vi "RT Main v0.82.vi"() -> ()   [LabVIEW 2017]
uses:
  Controls/Auto Delays.ctl
  support/Controls/All Inputs.ctl
  support/Controls/Index Details.ctl
  Global Variables/RT GV.vi
  support/Message Queue/Enqueue Message (Single).vi
  <vilib>/Utility/error.llb/Error Cluster From Error Code.vi
  <vilib>/rvi/errors/niLvFpgaAdjustHostInterfaceError.vi
  Global Variables/FPGA GV.vi
  Global Variables/Network Globals.vi
  <vilib>/FPGAPlugInAG/Dynamic/niLvFpga_Close_Dynamic.vi
  <vilib>/rvi/interface/nirviReadWriteControl/nirviReadWriteControl.xnode
  Controls/FPGA Ref.ctl
  <vilib>/rvi/interface/nirviCloseFPGA/nirviCloseFPGA.xnode
  support/Message Queue/Message Queue.lvlib
  NiFpgaLv.dll
  <vilib>/rvi/interface/Simulation/niFpgaSimulationCallBeginRW.vi
panel:
  in  "Auto Para":T1={"Agitator Delays"=[400, 250], "TF Delays"=[700, 800, 2], "Insertion Delays"=[100, 500], "Cutting Delays"=[300, 300, 100], "PF Delays"=[250, 30000], "Measur. Delays"=[500.0, 188.9, 1.0], "Reject Delays"=[500], "BF Delays"=[1000, 1000]}
  in  "Counts in":cluster{"OutputCount":u32, "RejectCount":u32}
  in  "Stop Button 4":bool
  in  "Stop Button 3":bool
  in  "Stop Button 2":bool
  out "error out":errorcluster
  out "Wrong Message":string
  in  "Stop Button":bool
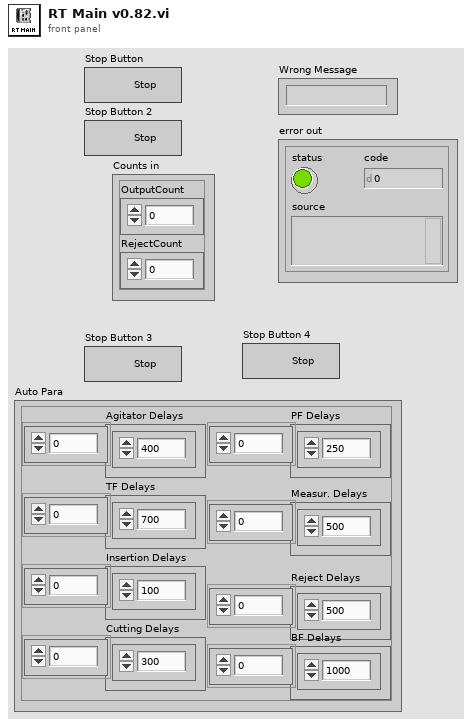
[diagram p1: front panel]
types:
  T1 = typedef "Auto Delays.ctl" = cluster{"Agitator Delays":u32[], "TF Delays":u32[], "Insertion Delays":u32[], "Cutting Delays":u32[], "PF Delays":u32[], "Measur. Delays":dbl[], "Reject Delays":u32[], "BF Delays":u32[]}
  T2 = typedef "FPGA Ref.ctl" = refnum<k20>
  T3 = cluster{"TL_Red":bool, "TL_Orange":bool, "TL_Green":bool, "TL_Buzzer":bool, "SOL_Index_Rotary_CW":bool, "SOL_Index_CNVR_Rotary_CCW":bool, "SOL_Index_CNVR_Stopper_Rear":bool, "SOL_Index_CNVR_Output _Separator _Rear":bool, "Bowl  Feeder_ ON":bool, "Pump_CNVR_Motor _ON":bool, "SOL_Gating_CYL_Rear":bool, "SOL_Tube_Feed_Agitatator":bool, "SOL_Tube_Feed_Gating_CYL":bool, "SOL_Insertion _CYL":bool, "SOL_Insertion_Clamp_CYL":bool, "SOL_Cutting_CYL":bool, "SOL_Cutting_Clamp_CYL":bool, "SOL_Insertion_Air_Nozzle":bool, "SOL_Measurement_CYL":bool, "SOL_Measure_Clamp_CYL":bool, "SOL_Rejection CYL_1":bool, "SOL_Rejection CYL_2":bool, "SOL_Rejection CYL_3":bool, "SOL_Rejection CYL_4":bool, "DO1.24":bool, "DO1.25":bool, "DO1.26":bool, "DO1.27":bool, "DO1.28":bool, "DO1.29":bool, "DO1.30":bool, "DO1.31":bool}
  T4 = typedef "All Inputs.ctl" = cluster{"DI 1":cluster{"Machine_ON":bool, "E_stop ":bool, "SW_Pressure":bool, "SW_Start ":bool, "SW_Reset":bool, "SW_Stop":bool, "SW_Door":bool, "RS_Index_Rotary_CW":bool, "RS_Index_Rotary_CCW":bool, "RS_Index_Stopper _Rear":bool, "RS_Index_Output_Separator_Rear":bool, "PES_Index_Pallet_Sensor":bool, "PES_Index_Output_Part Sensor":bool, "ICS_BF_Low_Level_1":bool, "ICS_BF_Low_Level_2":bool, "ICS_BF_Pump_CNVR_Full_1":bool, "ICS_BF_Pump_CNVR_Full_2":bool, "ICS_BF_Pump_CNVR_Full_3":bool, "ICS_BF_Pump_CNVR_Full_4":bool, "PES_PC_Pump Presence_1":bool, "PES_PC_Pump Presence_2":bool, "PES_PC_Pump Presence_3":bool, "PES_PC_Pump Presence_4":bool, "RS_PC_Gating_Front":bool, "PES_Pump_Interference":bool, "PES_TF_Low_Level":bool, "PES_Tube Presence_1":bool, "PES_Tube Presence_2":bool, "PES_Tube Presence_3":bool, "PES_Tube Presence_4":bool, "DI1.30":bool, "DI1.31":bool}, "DI 2":cluster{"RS_Agitatator_1_Rear ":bool, "RS_Agitatator_2_Rear ":bool, "RS_TF_Gating CYL_Rear":bool, "RS_Insertion_1_Rear":bool, "RS_Insertion_1_Front":bool, "RS_Insertion _2_Rear":bool, "RS_Insertion _2_Front":bool, "RS_Insertion _3_Rear":bool, "RS_Insertion _3_Front":bool, "RS_Insertion _4_Rear":bool, "RS_Insertion _4_Front":bool, "RS_Insertion_Clamp_Rear":bool, "RS_Cutting_Rear":bool, "RS_Cutting_Clamp _Rear":bool, "RS_Measurement_1_Rear":bool, "RS_Measurement_2_Rear":bool, "RS_Measurement_3_Rear":bool, "RS_Measurement_4_Rear":bool, "RS_Measure_Clamp_Rear":bool, "RS_Rejection_1_Rear":bool, "RS_Rejection_2_Rear":bool, "RS_Rejection_3_Rear":bool, "RS_Rejection_4_Rear":bool, "DI2.23":bool, "DI2.24":bool, "DI2.25":bool, "DI2.26":bool, "DI2.27":bool, "DI2.28":bool, "DI2.29":bool, "DI2.30":bool, "DI2.31":bool}, "IAS 1":dbl, "IAS 2":dbl, "IAS 3":dbl, "IAS 4":dbl, "DO 1":cluster{"TL_Red":bool, "TL_Orange":bool, "TL_Green":bool, "TL_Buzzer":bool, "SOL_Index_Rotary_CW":bool, "SOL_Index_CNVR_Rotary_CCW":bool, "SOL_Index_CNVR_Stopper_Rear":bool, "SOL_Index_CNVR_Output _Separator _Rear":bool, "Bowl  Feeder_ ON 1":bool, "Pump_CNVR_Motor _ON":bool, "SOL_PC_Gating_CYL_Rear":bool, "SOL_Tube_Feed_Agitatator":bool, "SOL_Tube_Feed_Gating_CYL":bool, "SOL_Insertion _CYL":bool, "SOL_Insertion_Clamp_CYL":bool, "SOL_Cutting_CYL":bool, "SOL_Cutting_Clamp_CYL":bool, "SOL_Insertion_Air_Nozzle":bool, "SOL_Measurement_CYL":bool, "DO1.19":bool, "SOL_Rejection CYL_1":bool, "SOL_Rejection CYL_2":bool, "SOL_Rejection CYL_3":bool, "SOL_Rejection CYL_4":bool, "Bowl  Feeder_ ON 2":bool, "SOL_BF_BlowerON":bool, "SOL_BF1_Track1":bool, "SOL_BF1_Track2":bool, "SOL_BF2_Track1":bool, "SOL_BF2_Track2":bool, "DO1.30":bool, "DO1.31":bool}}
  T5 = typedef "Index Details.ctl" = cluster{"Time (ms)":u32, "Waveform Graph":i16[]}
  T6 = cluster{T1, "Reject Pallets":cluster{"Reject 1":bool, "Reject 2":bool, "Reject 3":bool, "Reject 4":bool}}
  T7 = cluster{string, dbl, "Counts in":cluster{"OutputCount":u32, "RejectCount":u32}, "Auto Para":T1}
  T8 = cluster{"TL_Red":bool, "TL_Orange":bool, "TL_Green":bool, "TL_Buzzer":bool, "SOL_Index_Rotary_CW":bool, "SOL_Index_CNVR_Rotary_CCW":bool, "SOL_Index_CNVR_Stopper_Rear":bool, "SOL_Index_CNVR_Output _Separator _Rear":bool, "Bowl Feeder_ ON1":bool, "Pump_CNVR_Motor _ON":bool, "SOL_PC_Gating_CYL_Rear":bool, "SOL_Tube_Feed_Agitatator":bool, "SOL_Tube_Feed_Gating_CYL":bool, "SOL_Insertion _CYL":bool, "SOL_Insertion_Clamp_CYL":bool, "SOL_Cutting_CYL":bool, "SOL_Cutting_Clamp_CYL":bool, "SOL_Insertion_Air_Nozzle":bool, "SOL_Measurement_CYL":bool, "DO1.19":bool, "SOL_Rejection CYL_1":bool, "SOL_Rejection CYL_2":bool, "SOL_Rejection CYL_3":bool, "SOL_Rejection CYL_4":bool, "Bowl Feeder_ON2":bool, "SOL_BF_BlowerON":bool, "SOL_BF1_Track1":bool, "SOL_BF1_Track2":bool, "SOL_BF2_Track1":bool, "SOL_BF2_Track2":bool, "DO1.30":bool, "DO1.31":bool}
  T9 = cluster{"Machine_ON":bool, "E_stop ":bool, "SW_Pressure":bool, "SW_Start ":bool, "SW_Reset":bool, "SW_Stop":bool, "SW_Door":bool, "RS_Index_Rotary_CW":bool, "RS_Index_Rotary_CCW":bool, "RS_Index_Stopper _Rear":bool, "RS_Index_Output_Separator_Rear":bool, "PES_Index_Pallet_Sensor":bool, "PES_Index_Output_Part Sensor":bool, "ICS_BF_Low_Level_1":bool, "ICS_BF_Low_Level_2":bool, "ICS_BF_Pump_CNVR_Full_1":bool, "ICS_BF_Pump_CNVR_Full_2":bool, "ICS_BF_Pump_CNVR_Full_3":bool, "ICS_BF_Pump_CNVR_Full_4":bool, "PES_PC_Pump Presence_1":bool, "PES_PC_Pump Presence_2":bool, "PES_PC_Pump Presence_3":bool, "PES_PC_Pump Presence_4":bool, "RS_PC_Gating_Front":bool, "PES_Pump_Interference":bool, "PES_TF_Low_Level":bool, "PES_Tube Presence_1":bool, "PES_Tube Presence_2":bool, "PES_Tube Presence_3":bool, "PES_Tube Presence_4":bool, "DI1.30":bool, "DI1.31":bool}
  T10 = cluster{"RS_Agitatator_1_Rear ":bool, "RS_Agitatator_2_Rear ":bool, "RS_TF_Gating CYL_Rear":bool, "RS_Insertion_1_Rear":bool, "RS_Insertion_1_Front":bool, "RS_Insertion _2_Rear":bool, "RS_Insertion _2_Front":bool, "RS_Insertion _3_Rear":bool, "RS_Insertion _3_Front":bool, "RS_Insertion _4_Rear":bool, "RS_Insertion _4_Front":bool, "RS_Insertion_Clamp_Rear":bool, "RS_Cutting_Rear":bool, "RS_Cutting_Clamp _Rear":bool, "RS_Measurement_1_Rear":bool, "RS_Measurement_2_Rear":bool, "RS_Measurement_3_Rear":bool, "RS_Measurement_4_Rear":bool, "DI2.18":bool, "RS_Rejection_1_Rear":bool, "RS_Rejection_2_Rear":bool, "RS_Rejection_3_Rear":bool, "RS_Rejection_4_Rear":bool, "DI2.23":bool, "DI2.24":bool, "DI2.25":bool, "DI2.26":bool, "DI2.27":bool, "DI2.28":bool, "DI2.29":bool, "DI2.30":bool, "DI2.31":bool}
  T11 = cluster{"Measurements":cluster{"1":dbl, "2":dbl, "3":dbl, "4":dbl}, "Reject Pallets":cluster{"Reject 1":bool, "Reject 2":bool, "Reject 3":bool, "Reject 4":bool}}
  T12 = typedef "Auto Times.ctl" = cluster{"Index Time":u32, "TF Time":u32, "Insertion Time":u32, "Cutting Time":u32, "PF Time":u32, "Meas. Time":u32, "Reject Time":u32}
  T13 = cluster{"Auto Times":T12, "Results":cluster{"Measurements":cluster{"1":dbl, "2":dbl, "3":dbl, "4":dbl}, "Reject Pallets":cluster{"Reject 1":bool, "Reject 2":bool, "Reject 3":bool, "Reject 4":bool}}, "OutputCount":u32, "error out":errorcluster}
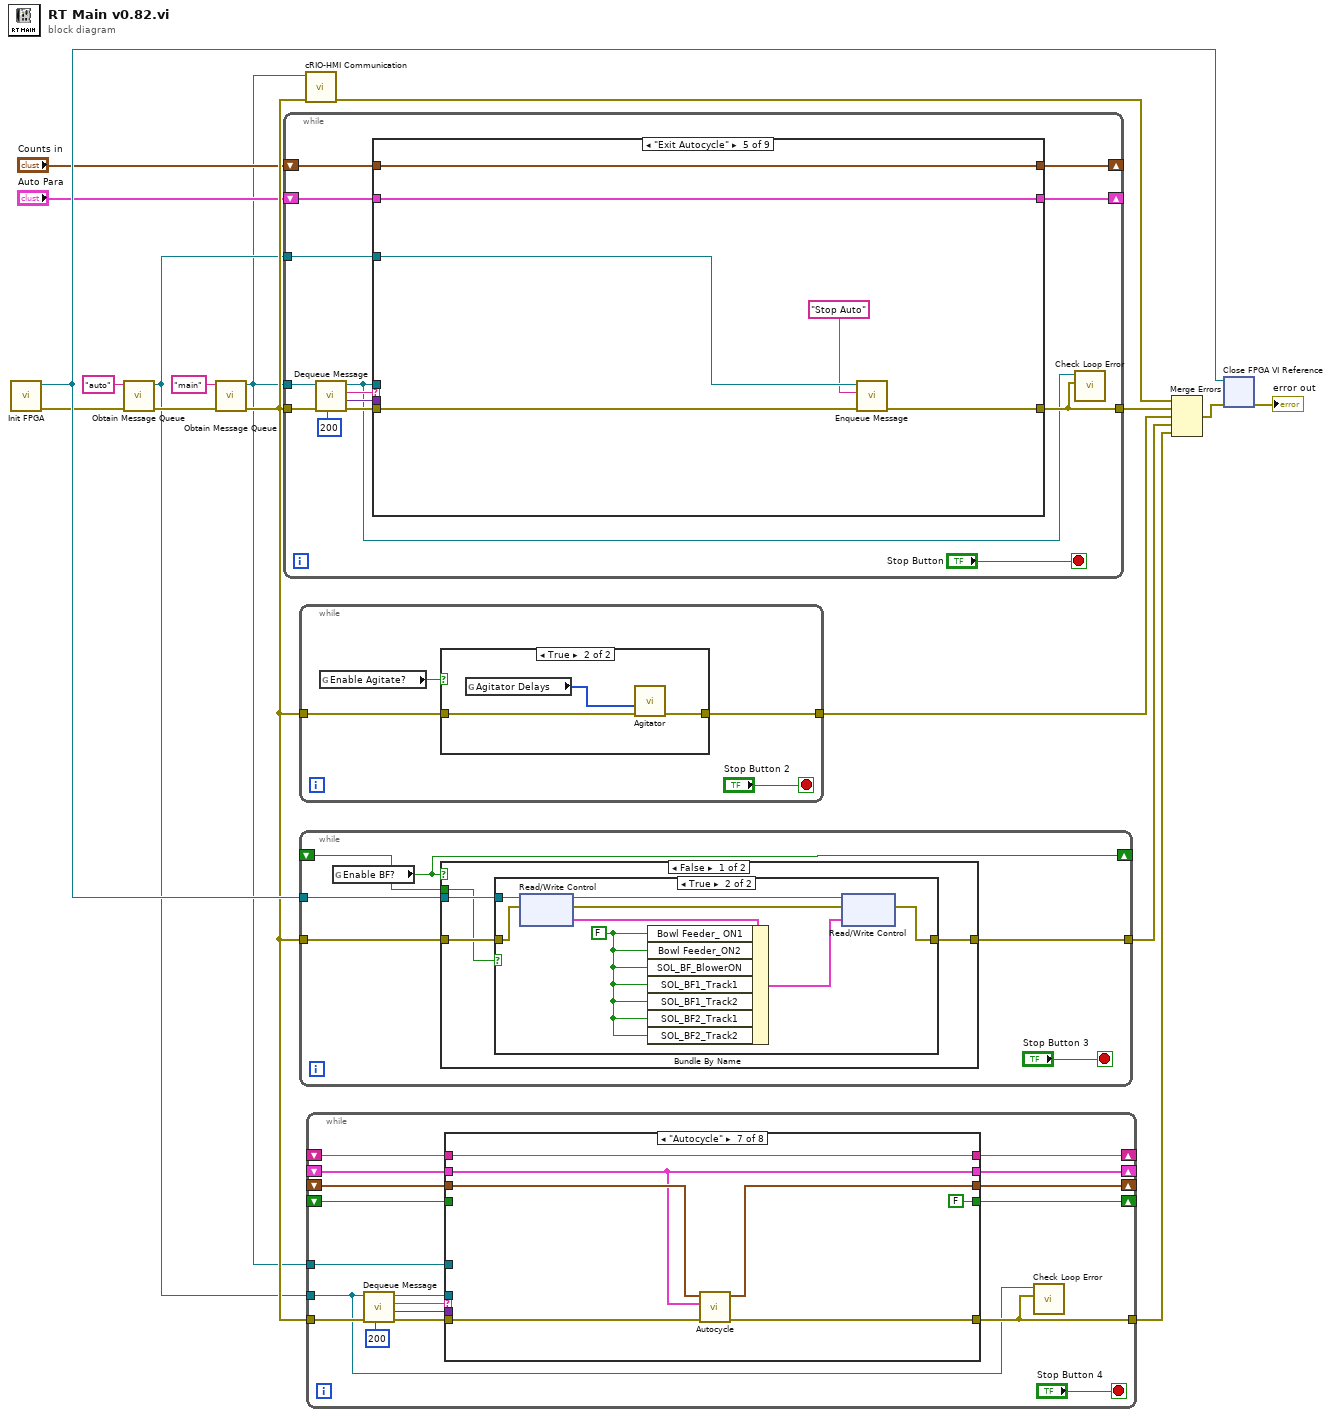
[diagram p0: block diagram]
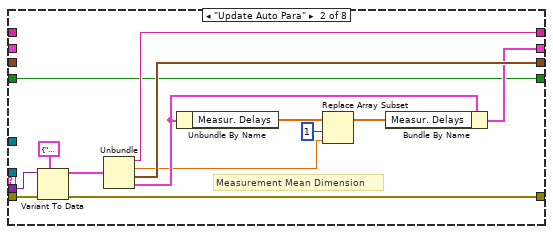
[diagram p3: hidden frame]
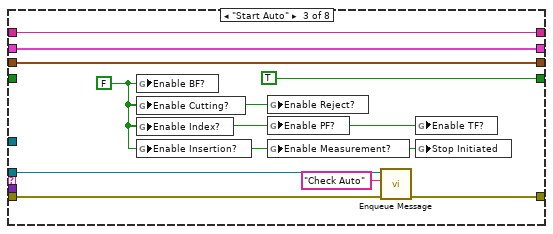
[diagram p4: hidden frame]
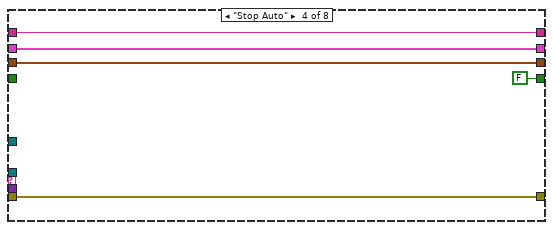
[diagram p5: hidden frame]
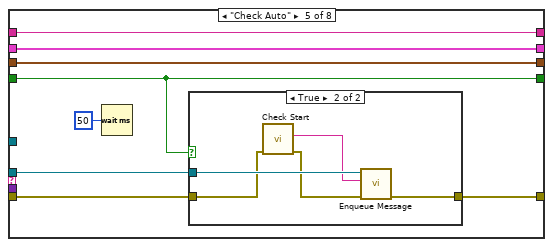
[diagram p6: hidden frame]
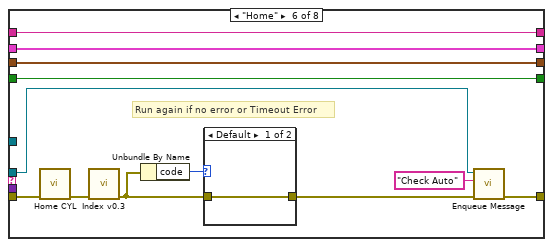
[diagram p8: hidden frame]
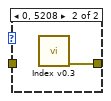
[diagram p9: hidden frame]
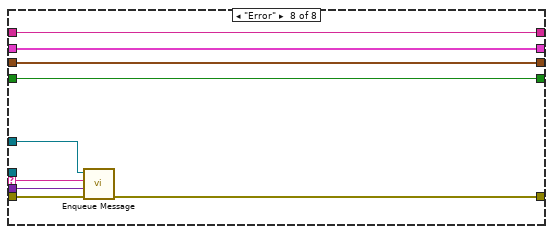
[diagram p10: hidden frame]
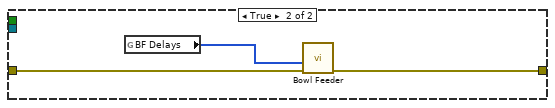
[diagram p12: hidden frame]
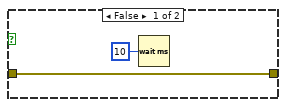
[diagram p13: hidden frame]
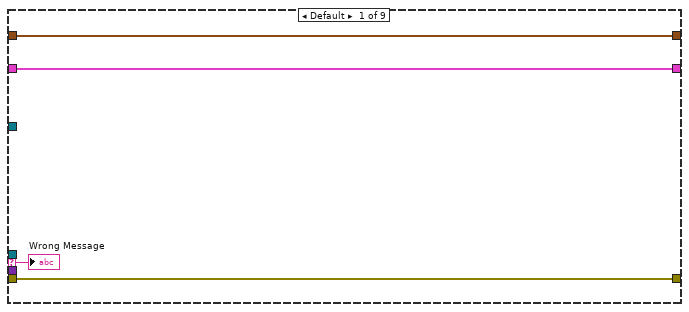
[diagram p14: hidden frame]
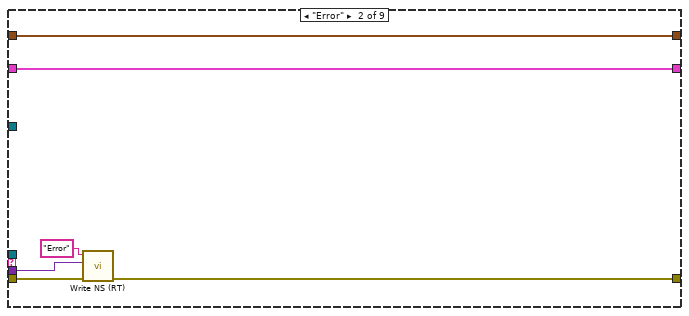
[diagram p15: hidden frame]
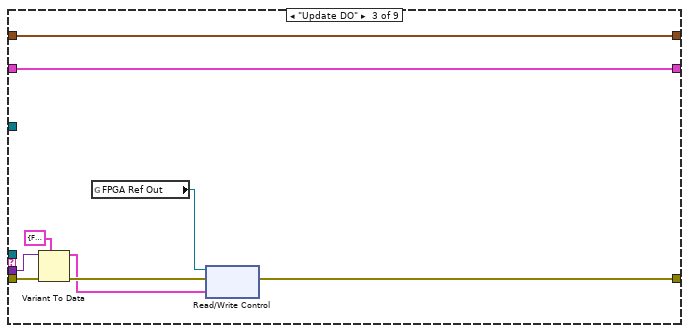
[diagram p16: hidden frame]
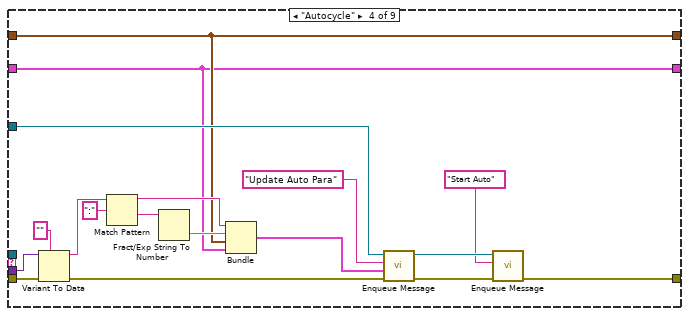
[diagram p17: hidden frame]
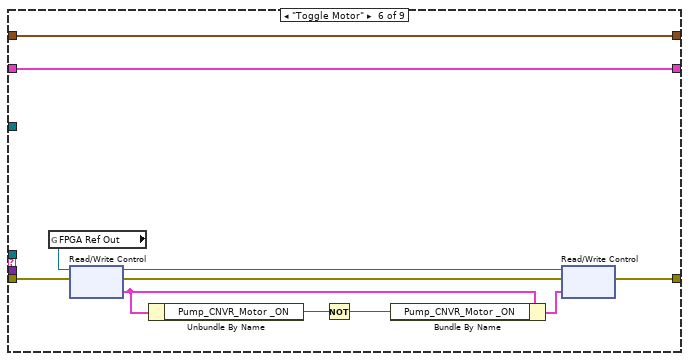
[diagram p18: hidden frame]
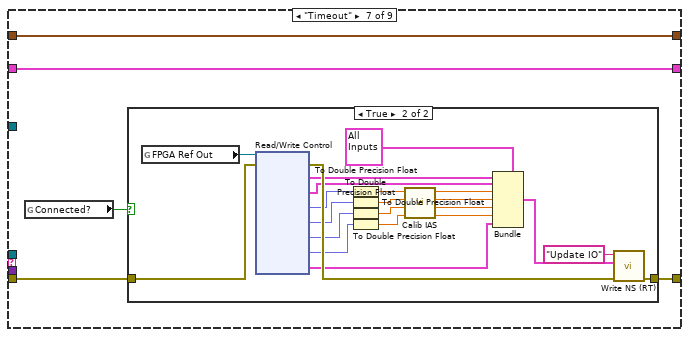
[diagram p19: hidden frame]
diagram:
  n1 = call "Init FPGA.vi"() -> ("error out"=w6:errorcluster, "FPGA Ref Out"=w11:T2)  [unwired: 10 in]
  n2 = call "Obtain Message Queue.vi"("error in (no error)"=w6, "name"="auto") -> ("error out"=w5:errorcluster, "Message Queue"=w2:refnum<queue>)  [unwired: 8 in]
  n3 = call "Obtain Message Queue.vi"("error in (no error)"=w5, "name"="main") -> ("error out"=w10:errorcluster, "Message Queue"=w1:refnum<queue>)  [unwired: 8 in]
  n4 = while {
    tunnel: w10 -> [w30]
    tunnel: w1 -> [w29]
    tunnel: [w25] -> w17
    tunnel: w2 -> [w22]
    shift-right: [w19] -> _
    shift-left: "Auto Para" -> [w20]
    shift-right: [w18] -> _
    shift-left: "Counts in" -> [w21]
    stop <- "Stop Button" stop-if-true
    n5 = call "Dequeue Message.vi"("timeout"=200, "error in (no error)"=w30, "Message Queue"=w29) -> ("error out"=w28:errorcluster, "Message Data"=w26:variant, "Message"=w27:string, "dup Message Queue"=w24:refnum<queue>)  [unwired: 5 in]
    n6 = case shown="\"Exit Autocycle\"" w27 {
      selector: w27 -> [w35 _ _ _ _ _ _ _ _]
      tunnel: w28 -> [w34 w39 w50 w68 w74 w84 w89 w125 w152]
      tunnel: w24 -> [_ _ _ _ _ _ _ w117 _]
      tunnel: w26 -> [_ w37 w49 w67 _ _ _ _ w151]
      tunnel: [w34 w38 w45 w53 w70 w82 w90 w118 w147] -> w25
      tunnel: w22 -> [_ _ _ w60 w73 _ _ _ _]
      tunnel: w21 -> [w33 w41 w43 w57 w72 w76 w87 w114 w138]
      tunnel: w20 -> [w32 w40 w42 w56 w71 w75 w86 w115 w137]
      tunnel: [w32 w40 w42 w56 w71 w75 w86 w115 w137] -> w19
      tunnel: [w33 w41 w43 w57 w72 w76 w87 w114 w138] -> w18
      frame Default {
        "Wrong Message" <- w35
      }
      frame "Error" {
        n7 = call "Write NS (RT).vi"("error in (no error)"=w39, "Message Data"=w37, "Message"="Error") -> ("error out"=w38:errorcluster)  [unwired: 8 in]
      }
      frame "Update DO" {
        n8 = Variant To Data(error in=w50, type=T3 {"TL_Red"=FALSE, "TL_Orange"=FALSE, "TL_Green"=FALSE, "TL_Buzzer"=FALSE, "SOL_Index_Rotary_CW"=FALSE, "SOL_Index_CNVR_Rotary_CCW"=FALSE, "SOL_Index_CNVR_Stopper_Rear"=FALSE, "SOL_Index_CNVR_Output _Separator _Rear"=FALSE, "Bowl  Feeder_ ON"=FALSE, "Pump_CNVR_Motor _ON"=FALSE, "SOL_Gating_CYL_Rear"=FALSE, "SOL_Tube_Feed_Agitatator"=FALSE, "SOL_Tube_Feed_Gating_CYL"=FALSE, "SOL_Insertion _CYL"=FALSE, "SOL_Insertion_Clamp_CYL"=FALSE, "SOL_Cutting_CYL"=FALSE, "SOL_Cutting_Clamp_CYL"=FALSE, "SOL_Insertion_Air_Nozzle"=FALSE, "SOL_Measurement_CYL"=FALSE, "SOL_Measure_Clamp_CYL"=FALSE, "SOL_Rejection CYL_1"=FALSE, "SOL_Rejection CYL_2"=FALSE, "SOL_Rejection CYL_3"=FALSE, "SOL_Rejection CYL_4"=FALSE, "DO1.24"=FALSE, "DO1.25"=FALSE, "DO1.26"=FALSE, "DO1.27"=FALSE, "DO1.28"=FALSE, "DO1.29"=FALSE, "DO1.30"=FALSE, "DO1.31"=FALSE} ("DO 1"), Variant=w49) -> (data=w44:T3, error out=w46:errorcluster)
        n9 = global read "FPGA GV.vi" "FPGA Ref Out"() -> (w47:T2)
        n10 = xnode "Read/Write Control"("FPGA VI Reference In"=w47, "error in"=w46, "DO 1"=w44) -> ("error out"=w45:errorcluster)  [unwired: 1 out]
      }
      frame "Autocycle" {
        n11 = Variant To Data(error in=w68, type="", Variant=w67) -> (data=w63:string, error out=w61:errorcluster)
        n12 = Match Pattern(string=w63, regular expression=":") -> (before substring=w59:string, after substring=w64:string)  [unwired: 1 in, 2 out]
        n13 = Fract/Exp String To Number(string=w64) -> (number=w58:dbl)  [unwired: 3 in, 1 out]
        n14 = Bundle(w59, w58, "Counts in"=w57, "Auto Para"=w56) -> (w55:T7)  [unwired: 1 in]
        n15 = call-poly "Enqueue Message.vi"("error in (no error)"=w61, "Message Data"=w55, "Message"="Update Auto Para", "Message Queue"=w60) -> ("error out"=w54:errorcluster, "dup Message Queue"=w52:refnum<queue>)  [unwired: 6 in]
        n16 = call-poly "Enqueue Message.vi"("error in (no error)"=w54, "Message"="Start Auto", "Message Queue"=w52) -> ("error out"=w53:errorcluster)  [unwired: 7 in, 1 out]
      }
      frame "Exit Autocycle" {
        n17 = call-poly "Enqueue Message.vi"("error in (no error)"=w74, "Message"="Stop Auto", "Message Queue"=w73) -> ("error out"=w70:errorcluster)  [unwired: 7 in, 1 out]
      }
      frame "Toggle Motor" {
        n18 = global read "FPGA GV.vi" "FPGA Ref Out"() -> (w85:T2)
        n19 = xnode "Read/Write Control"("FPGA VI Reference In"=w85, "error in"=w84) -> ("FPGA VI Reference Out"=w81:T2, "error out"=w83:errorcluster, "DO 1"=w79:T8)
        n20 = Unbundle By Name(w79) -> ("Pump_CNVR_Motor _ON"=w80:bool)
        n21 = Not(x=w80) -> (.not. x?=w77:bool)
        n22 = Bundle By Name(cluster=w79, "Pump_CNVR_Motor _ON"=w77) -> (w78:T8)
        n23 = xnode "Read/Write Control"("FPGA VI Reference In"=w81, "error in"=w83, "DO 1"=w78) -> ("error out"=w82:errorcluster)  [unwired: 1 out]
      }
      frame "Timeout" {
        n24 = global read "Network Globals.vi" "Connected?"() -> (w88:bool)
        n25 = case shown="True" w88 {
          tunnel: [w91 w112] -> w90
          tunnel: w89 -> [w91 w110]
          frame False {
          }
          frame True {
            n26 = global read "FPGA GV.vi" "FPGA Ref Out"() -> (w111:T2)
            n27 = xnode "Read/Write Control"("FPGA VI Reference In"=w111, "error in"=w110) -> ("error out"=w109:errorcluster, "DI 1"=w108:T9, "DI 2"=w107:T10, "AI0"=w106:fxp<+/-,27,6>, "AI1"=w105:fxp<+/-,27,6>, "AI2"=w104:fxp<+/-,27,6>, "AI3"=w103:fxp<+/-,27,6>, "DO 1"=w100:T8)  [unwired: 1 out]
            n28 = To Double Precision Float(number=w106) -> (double precision float=w93:dbl)
            n29 = To Double Precision Float(number=w105) -> (double precision float=w95:dbl)
            n30 = To Double Precision Float(number=w104) -> (double precision float=w97:dbl)
            n31 = To Double Precision Float(number=w103) -> (double precision float=w99:dbl)
            n32 = call "Calib IAS.vi"("x 4"=w99, "x 3"=w97, "x 2"=w95, "x"=w93) -> ("y 4"=w98:dbl, "y 3"=w96:dbl, "y 2"=w94:dbl, "y 1"=w92:dbl)  [unwired: 4 in]
            n33 = Bundle(cluster=T4 {"DI 1"={"Machine_ON"=FALSE, "E_stop "=FALSE, "SW_Pressure"=FALSE, "SW_Start "=FALSE, "SW_Reset"=FALSE, "SW_Stop"=FALSE, "SW_Door"=FALSE, "RS_Index_Rotary_CW"=FALSE, "RS_Index_Rotary_CCW"=FALSE, "RS_Index_Stopper _Rear"=FALSE, "RS_Index_Output_Separator_Rear"=FALSE, "PES_Index_Pallet_Sensor"=FALSE, "PES_Index_Output_Part Sensor"=FALSE, "ICS_BF_Low_Level_1"=FALSE, "ICS_BF_Low_Level_2"=FALSE, "ICS_BF_Pump_CNVR_Full_1"=FALSE, "ICS_BF_Pump_CNVR_Full_2"=FALSE, "ICS_BF_Pump_CNVR_Full_3"=FALSE, "ICS_BF_Pump_CNVR_Full_4"=FALSE, "PES_PC_Pump Presence_1"=FALSE, "PES_PC_Pump Presence_2"=FALSE, "PES_PC_Pump Presence_3"=FALSE, "PES_PC_Pump Presence_4"=FALSE, "RS_PC_Gating_Front"=FALSE, "PES_Pump_Interference"=FALSE, "PES_TF_Low_Level"=FALSE, "PES_Tube Presence_1"=FALSE, "PES_Tube Presence_2"=FALSE, "PES_Tube Presence_3"=FALSE, "PES_Tube Presence_4"=FALSE, "DI1.30"=FALSE, "DI1.31"=FALSE}, "DI 2"={"RS_Agitatator_1_Rear "=FALSE, "RS_Agitatator_2_Rear "=FALSE, "RS_TF_Gating CYL_Rear"=FALSE, "RS_Insertion_1_Rear"=FALSE, "RS_Insertion_1_Front"=FALSE, "RS_Insertion _2_Rear"=FALSE, "RS_Insertion _2_Front"=FALSE, "RS_Insertion _3_Rear"=FALSE, "RS_Insertion _3_Front"=FALSE, "RS_Insertion _4_Rear"=FALSE, "RS_Insertion _4_Front"=FALSE, "RS_Insertion_Clamp_Rear"=FALSE, "RS_Cutting_Rear"=FALSE, "RS_Cutting_Clamp _Rear"=FALSE, "RS_Measurement_1_Rear"=FALSE, "RS_Measurement_2_Rear"=FALSE, "RS_Measurement_3_Rear"=FALSE, "RS_Measurement_4_Rear"=FALSE, "RS_Measure_Clamp_Rear"=FALSE, "RS_Rejection_1_Rear"=FALSE, "RS_Rejection_2_Rear"=FALSE, "RS_Rejection_3_Rear"=FALSE, "RS_Rejection_4_Rear"=FALSE, "DI2.23"=FALSE, "DI2.24"=FALSE, "DI2.25"=FALSE, "DI2.26"=FALSE, "DI2.27"=FALSE, "DI2.28"=FALSE, "DI2.29"=FALSE, "DI2.30"=FALSE, "DI2.31"=FALSE}, "IAS 1"=0.0, "IAS 2"=0.0, "IAS 3"=0.0, "IAS 4"=0.0, "DO 1"={"TL_Red"=FALSE, "TL_Orange"=FALSE, "TL_Green"=FALSE, "TL_Buzzer"=FALSE, "SOL_Index_Rotary_CW"=FALSE, "SOL_Index_CNVR_Rotary_CCW"=FALSE, "SOL_Index_CNVR_Stopper_Rear"=FALSE, "SOL_Index_CNVR_Output _Separator _Rear"=FALSE, "Bowl  Feeder_ ON 1"=FALSE, "Pump_CNVR_Motor _ON"=FALSE, "SOL_PC_Gating_CYL_Rear"=FALSE, "SOL_Tube_Feed_Agitatator"=FALSE, "SOL_Tube_Feed_Gating_CYL"=FALSE, "SOL_Insertion _CYL"=FALSE, "SOL_Insertion_Clamp_CYL"=FALSE, "SOL_Cutting_CYL"=FALSE, "SOL_Cutting_Clamp_CYL"=FALSE, "SOL_Insertion_Air_Nozzle"=FALSE, "SOL_Measurement_CYL"=FALSE, "DO1.19"=FALSE, "SOL_Rejection CYL_1"=FALSE, "SOL_Rejection CYL_2"=FALSE, "SOL_Rejection CYL_3"=FALSE, "SOL_Rejection CYL_4"=FALSE, "Bowl  Feeder_ ON 2"=FALSE, "SOL_BF_BlowerON"=FALSE, "SOL_BF1_Track1"=FALSE, "SOL_BF1_Track2"=FALSE, "SOL_BF2_Track1"=FALSE, "SOL_BF2_Track2"=FALSE, "DO1.30"=FALSE, "DO1.31"=FALSE}}, "DI 1"=w108, "DI 2"=w107, "IAS 1"=w92, "IAS 2"=w94, "IAS 3"=w96, "IAS 4"=w98, "DO 1"=w100) -> (w102:T4)
            n34 = call "Write NS (RT).vi"("error in (no error)"=w109, "Message Data"=w102, "Message"="Update IO") -> ("error out"=w112:errorcluster)  [unwired: 8 in]
          }
        }
      }
      frame "Manual Index" {
        n35 = call "Index v0.3.vi"("error in (no error)"=w125) -> ("error out"=w123:errorcluster, "Waveform Graph"=w121:i16[], "Index Time"=w122:u32)  [unwired: 7 in, 1 out]
        n36 = Bundle(cluster=T5 {"Time (ms)"=0, "Waveform Graph"=[]}, "Time (ms)"=w122, "Waveform Graph"=w121) -> (w120:T5)
        n37 = call "Write NS (RT).vi"("error in (no error)"=w123, "Message Data"=w120, "Message"="Update Index") -> ("error out"=w119:errorcluster)  [unwired: 8 in]
        n38 = flat-sequence {
          tunnel: w119 -> [w129]
          tunnel: [w128] -> w118
          tunnel: w117 -> [w126]
          frame #0 {
            n39 = global read "RT GV.vi" "Continuous Index?"() -> (w127:bool)
            n40 = case shown="True" w127 {
              tunnel: w129 -> [w130 w134]
              tunnel: [w130 w133] -> w128
              tunnel: w126 -> [_ w131]
              frame False {
              }
              frame True {
                n41 = call-poly "Enqueue Message.vi"("error in (no error)"=w134, "Message"="Manual Index", "Message Queue"=w131) -> ("error out"=w133:errorcluster)  [unwired: 7 in, 1 out]
              }
            }
          }
        }
      }
      frame "Manual Run" {
        n42 = Variant To Data(error in=w152, type=T6 {{"Agitator Delays"=[1000], "TF Delays"=[1000], "Insertion Delays"=[1000], "Cutting Delays"=[1000], "PF Delays"=[1000], "Measur. Delays"=[1000.0], "Reject Delays"=[1000], "BF Delays"=[1000]}, "Reject Pallets"={"Reject 1"=FALSE, "Reject 2"=FALSE, "Reject 3"=FALSE, "Reject 4"=FALSE}}, Variant=w151) -> (data=w143:T6, error out=w150:errorcluster)
        n43 = Unbundle(w143) -> (w140:T1)  [unwired: 1 out]
        n44 = Unbundle By Name(w140) -> ("Agitator Delays"=w136:u32[], "BF Delays"=w135:u32[])
        n45 = call "Manual.vi"("error in"=w150, "Auto Delays"=w140) -> ("error out"=w142:errorcluster, "OutputCount"=w141:u32, "Results"=w139:T11, "Auto Times"=w146:T12)  [unwired: 6 in]
        n46 = global write "RT GV.vi" "Agitator Delays"(w136) -> ()
        n47 = global write "RT GV.vi" "BF Delays"(w135) -> ()
        n48 = Bundle("Auto Times"=w146, "Results"=w139, "OutputCount"=w141, "error out"=w142) -> (w145:T13)  [unwired: 1 in]
        n49 = call "Write NS (RT).vi"("Message Data"=w145, "Message"="Manual Status") -> ("error out"=w148:errorcluster)  [unwired: 9 in]
        n50 = Merge Errors(w148) -> (w147:errorcluster)
      }
    }
    n51 = call "Check Loop Error.vi"("error to process"=w25, "Message Queue"=w24) -> ()  [unwired: 8 in, 2 out]
  }
  n52 = while {
    tunnel: w10 -> [w156]
    tunnel: [w153] -> w13
    stop <- "Stop Button 2" stop-if-true
    n53 = global read "RT GV.vi" "Enable Agitate?"() -> (w155:bool)
    n54 = case shown="True" w155 {
      tunnel: w156 -> [w158 w161]
      tunnel: [w158 w160] -> w153
      frame False {
        n55 = Wait (ms)(milliseconds to wait=u32 10) -> ()  [unwired: 1 out]
      }
      frame True {
        n56 = global read "RT GV.vi" "Agitator Delays"() -> (w159:u32[])
        n57 = call "Agitator.vi"("error in (no error)"=w161, "Agitator Delays"=w159) -> ("error out"=w160:errorcluster)  [unwired: 8 in, 1 out]
      }
    }
  }
  n58 = while {
    tunnel: w10 -> [w167]
    tunnel: [w165] -> w12
    shift-right: [w164] -> _
    shift-left: _ -> [w163]
    tunnel: w11 -> [w162]
    stop <- "Stop Button 3" stop-if-true
    n59 = global read "RT GV.vi" "Enable BF?"() -> (w164:bool)
    n60 = case shown="False" w164 {
      tunnel: w167 -> [w171 w183]
      tunnel: [w170 w182] -> w165
      tunnel: w163 -> [w168 _]
      tunnel: w162 -> [w169 _]
      frame False {
        n61 = case shown="True" w168 {
          tunnel: w171 -> [w172 w175]
          tunnel: [w172 w174] -> w170
          tunnel: w169 -> [_ w173]
          frame False {
          }
          frame True {
            w176 = FALSE ("SOL_Index_Rotary_CW")
            n62 = xnode "Read/Write Control"("FPGA VI Reference In"=w173, "error in"=w175) -> ("FPGA VI Reference Out"=w177:T2, "error out"=w178:errorcluster, "DO 1"=w179:T8)
            n63 = Bundle By Name(cluster=w179, "Bowl Feeder_ ON1"=w176, "Bowl Feeder_ON2"=w176, "SOL_BF_BlowerON"=w176, "SOL_BF1_Track1"=w176, "SOL_BF1_Track2"=w176, "SOL_BF2_Track1"=w176, "SOL_BF2_Track2"=w176) -> (w180:T8)
            n64 = xnode "Read/Write Control"("FPGA VI Reference In"=w177, "error in"=w178, "DO 1"=w180) -> ("error out"=w174:errorcluster)  [unwired: 1 out]
          }
        }
      }
      frame True {
        n65 = global read "RT GV.vi" "BF Delays"() -> (w181:u32[])
        n66 = call "Bowl Feeder.vi"("error in (no error)"=w183, "BF Delays"=w181) -> ("error out"=w182:errorcluster)  [unwired: 8 in, 1 out]
      }
    }
  }
  n67 = call "cRIO-HMI Communication.vi"("error in (no error)"=w10, "Message Queue"=w1) -> ("error out"=w16:errorcluster)  [unwired: 9 in]
  n68 = while {
    tunnel: w10 -> [w197]
    tunnel: [w195] -> w9
    shift-right: [w199] -> _
    shift-left: _ -> [w200]
    tunnel: w2 -> [w187]
    shift-right: [w191] -> _
    shift-left: _ -> [w190]
    shift-right: [w189] -> _
    shift-left: _ -> [w188]
    shift-right: [w186] -> _
    shift-left: _ -> [w185]
    tunnel: w1 -> [w184]
    stop <- "Stop Button 4" stop-if-true
    n69 = call "Dequeue Message.vi"("timeout"=200, "error in (no error)"=w197, "Message Queue"=w187) -> ("error out"=w196:errorcluster, "Message Data"=w192:variant, "Message"=w193:string, "dup Message Queue"=w194:refnum<queue>)  [unwired: 5 in]
    n70 = case shown="\"Autocycle\"" w193 {
      selector: w193 -> [_ _ _ _ _ _ _ w274]
      tunnel: w196 -> [w206 w220 w225 w231 w237 w256 w269 w272]
      tunnel: [w206 w219 w224 w231 w239 w251 w268 w271] -> w195
      tunnel: w200 -> [w205 _ w229 w234 w242 w260 w267 w278]
      tunnel: [w205 w214 w229 w234 w242 w260 w266 w278] -> w199
      tunnel: w194 -> [_ _ w223 _ w238 w249 _ _]
      tunnel: w192 -> [_ w218 _ _ _ _ _ w273]
      tunnel: [w204 w215 w228 w233 w241 w259 w265 w277] -> w191
      tunnel: w190 -> [w204 _ w228 w233 w241 w259 w265 w277]
      tunnel: [w203 w208 w227 w232 w240 w258 w263 w276] -> w189
      tunnel: w188 -> [w203 _ w227 w232 w240 w258 w263 w276]
      tunnel: [w202 w207 TRUE FALSE w236 w257 FALSE w275] -> w186
      tunnel: w185 -> [w202 w207 _ _ w236 w257 _ w275]
      tunnel: w184 -> [_ _ _ _ _ _ _ w270]
      frame Default {
      }
      frame "Update Auto Para" {
        # "Measurement Mean Dimension"
        n71 = Variant To Data(error in=w220, type=T7 {"", 0.0, "Counts in"={"OutputCount"=0, "RejectCount"=0}, "Auto Para"={"Agitator Delays"=[], "TF Delays"=[], "Insertion Delays"=[], "Cutting Delays"=[], "PF Delays"=[], "Measur. Delays"=[], "Reject Delays"=[], "BF Delays"=[]}} ("cluster"), Variant=w218) -> (data=w216:T7, error out=w219:errorcluster)
        n72 = Unbundle(w216) -> (w215:string, w210:dbl, "Counts in"=w214:cluster{"OutputCount":u32, "RejectCount":u32}, "Auto Para"=w213:T1)
        n73 = Unbundle By Name(w213) -> ("Measur. Delays"=w212:dbl[])
        n74 = Replace Array Subset(array=w212, new element=w210, index=1) -> (w209:dbl[])
        n75 = Bundle By Name(cluster=w213, "Measur. Delays"=w209) -> (w208:T1)
      }
      frame "Start Auto" {
        w221 = FALSE ("Enable BF?")
        n76 = global write "RT GV.vi" "Enable BF?"(w221) -> ()
        n77 = global write "RT GV.vi" "Enable Cutting?"(w221) -> ()
        n78 = global write "RT GV.vi" "Enable Index?"(w221) -> ()
        n79 = global write "RT GV.vi" "Enable Insertion?"(w221) -> ()
        n80 = global write "RT GV.vi" "Enable Reject?"(w221) -> ()
        n81 = global write "RT GV.vi" "Enable PF?"(w221) -> ()
        n82 = global write "RT GV.vi" "Enable Measurement?"(w221) -> ()
        n83 = call-poly "Enqueue Message.vi"("error in (no error)"=w225, "Message"="Check Auto", "Message Queue"=w223) -> ("error out"=w224:errorcluster)  [unwired: 7 in, 1 out]
        n84 = global write "RT GV.vi" "Enable TF?"(w221) -> ()
        n85 = global write "RT GV.vi" "Stop Initiated"(w221) -> ()
      }
      frame "Stop Auto" {
      }
      frame "Check Auto" {
        n86 = Wait (ms)(milliseconds to wait=u32 50) -> ()  [unwired: 1 out]
        n87 = case shown="True" w236 {
          tunnel: [w243 w248] -> w239
          tunnel: w238 -> [_ w247]
          tunnel: w237 -> [w243 w246]
          frame False {
          }
          frame True {
            n88 = call "Check Start.vi"("error in"=w246) -> ("error out"=w245:errorcluster, "Message"=w244:string)  [unwired: 9 in]
            n89 = call-poly "Enqueue Message.vi"("error in (no error)"=w245, "Message"=w244, "Message Queue"=w247) -> ("error out"=w248:errorcluster)  [unwired: 7 in, 1 out]
          }
        }
      }
      frame "Home" {
        # "Run again if no error or Timeout Error"
        n90 = call "Home CYL.vi"("error in"=w256) -> ("error out"=w255:errorcluster)  [unwired: 10 in]
        n91 = call "Index v0.3.vi"("error in (no error)"=w255) -> ("error out"=w253:errorcluster)  [unwired: 7 in, 3 out]
        n92 = Unbundle By Name(w253) -> ("code"=w254:i32)
        n93 = case shown="Default" w254 {
          tunnel: [w261 w262] -> w250
          tunnel: w253 -> [w261 _]
          frame Default {
          }
          frame 0, 5208 {
            n94 = call "Index v0.3.vi"() -> ("error out"=w262:errorcluster)  [unwired: 8 in, 3 out]
          }
        }
        n95 = call-poly "Enqueue Message.vi"("error in (no error)"=w250, "Message"="Check Auto", "Message Queue"=w249) -> ("error out"=w251:errorcluster)  [unwired: 7 in, 1 out]
      }
      frame "Autocycle" {
        n96 = call "Autocycle.vi"("error in"=w269, "Auto Para"=w263, "Counts in"=w267) -> ("error out"=w268:errorcluster, "Counts out"=w266:cluster{"OutputCount":u32, "RejectCount":u32})  [unwired: 7 in]
      }
      frame "Error" {
        n97 = call-poly "Enqueue Message.vi"("error in (no error)"=w272, "Message Data"=w273, "Message"=w274, "Message Queue"=w270) -> ("error out"=w271:errorcluster)  [unwired: 6 in, 1 out]
      }
    }
    n98 = call "Check Loop Error.vi"("error to process"=w195, "Message Queue"=w187) -> ()  [unwired: 8 in, 2 out]
  }
  n99 = Merge Errors(w16, w17, w13, w12, w9) -> (w15:errorcluster)
  n100 = xnode ("Close FPGA VI Reference")("FPGA VI Reference In"=w11, "error in"=w15) -> ("error out"=→"error out":errorcluster)
